vi "Init Serial.vi"(8 "error in (no error)":errorcluster, 10 "Baud (115200)":u32=115200, 11 "VISA resource name in":refnum<visa-resource-name>) -> (0 "error out":errorcluster, 2 "Identity":T1, 3 "VISA resource name Out":refnum<visa-resource-name>)   [LabVIEW 2024, in "CTIPicoVISA.lvlib"]
uses:
  CTIPicoVISA.lvlib
  <vilib>/Instr/_visa.llb/VISA Open Access Mode.ctl
  <vilib>/Instr/_visa.llb/VISA Configure Serial Port (Instr).vi
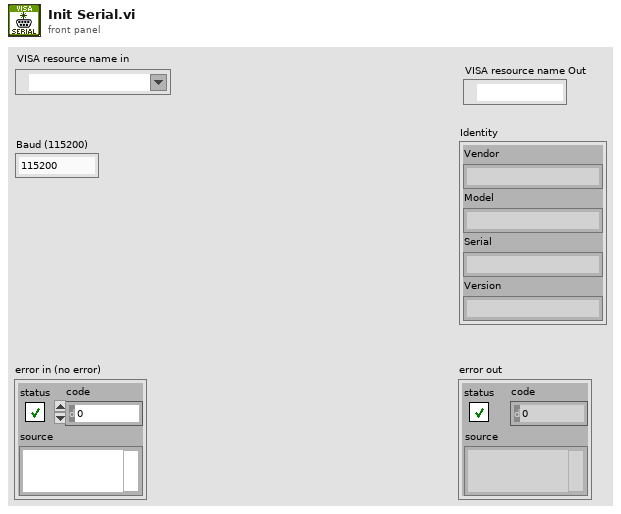
[diagram p1: front panel]
types:
  T1 = cluster{"Vendor":string, "Model":string, "Serial":string, "Version":string}
  T2 = typedef "VISA Open Access Mode.ctl" = u32
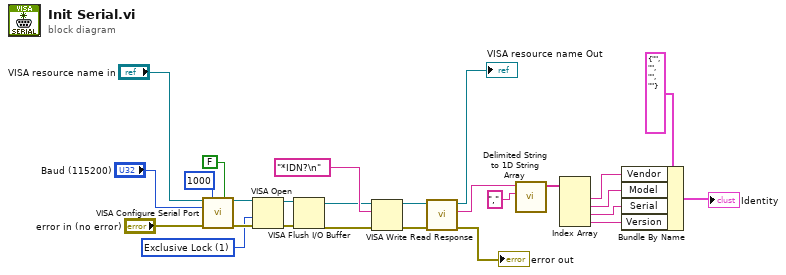
[diagram p0: block diagram]
diagram:
  w22 = T2 1 items=["VISA Defaults"=0, "Exclusive Lock"=1, "Load Configured Settings"=4] ("Access Mode")
  n1 = call-poly "VISA Configure Serial Port"("VISA resource name"="VISA resource name in", "timeout (10sec)"=u32 1000, "Enable Termination\nChar (T)"=FALSE ("Enable Termination\nChar (T)"), "baud rate (9600)"="Baud (115200)", "error in (no error)"="error in (no error)") -> ("VISA resource name out"=w23:refnum<visa-resource-name>, "error out"=w24:errorcluster)  [unwired: 9 in]
  n2 = VISA Open(access mode=w22, error in (no error)=w24, VISA resource name=w23) -> (VISA resource name=w21:refnum<visa-resource-name>, error out=w20:errorcluster)  [unwired: 2 in]
  n3 = VISA Flush I/O Buffer(VISA resource name=w21, error in (no error)=w20) -> (VISA resource name out=w14:refnum<visa-resource-name>, error out=w16:errorcluster)  [unwired: 1 in]
  n4 = VISA Write(VISA resource name=w14, write buffer="*IDN?\n", error in (no error)=w16) -> (VISA resource name out=w13:refnum<visa-resource-name>, error out=w12:errorcluster)  [unwired: 1 out]
  n5 = call "Read Response.vi"("error in (no error)"=w12, "VISA resource name"=w13) -> ("error out"=→"error out":errorcluster, "Response"=w5:string, "VISA resource name Out"=→"VISA resource name Out":refnum<visa-resource-name>)  [unwired: 6 in, 1 out]
  n6 = call <vilib>:"Delimited String to 1D String Array.vi"("delimiter"=",", "delimited string"=w5) -> ("string array"=w10:string[])  [unwired: 9 in]
  n7 = Index Array(array=w10) -> (element #1=w9:string, element #2=w8:string, element #3=w7:string, element #4=w6:string)  [unwired: 4 in]
  n8 = Bundle By Name(cluster=T1 {"Vendor"="", "Model"="", "Serial"="", "Version"=""} ("Identity"), "Vendor"=w9, "Model"=w8, "Serial"=w7, "Version"=w6) -> (→"Identity":T1)
